vi "Untitled 2.vi"() -> ()   [LabVIEW 2013, in "Generic Data Logger.lvlib"]
uses:
  Generic Data Logger.lvlib
panel:
  out "return count":u32
  out "error out":errorcluster
  out "find list":string[](array[string])
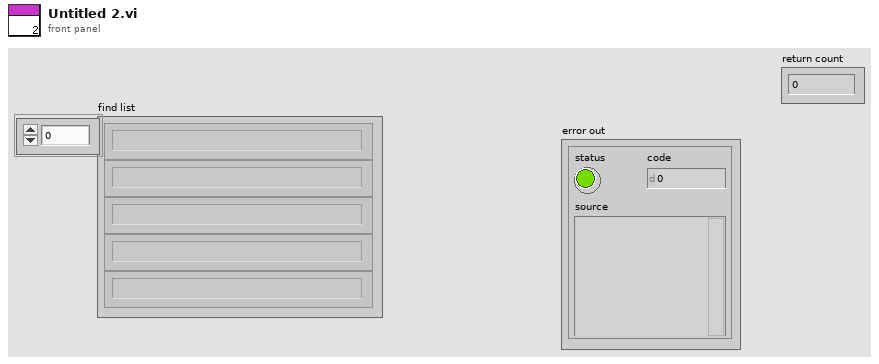
[diagram p1: front panel]
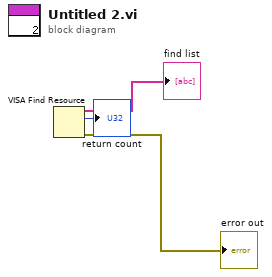
[diagram p0: block diagram]
diagram:
  n1 = VISA Find Resource() -> (0:→"error out":errorcluster, 2:→"return count":u32, 3:→"find list":string[])  [unwired: 3 in]
